vi "Example.vi"() -> ()   [LabVIEW 2014, in "Vaisala Library.lvlib" / "Vaisala.lvclass"]
doc: "Simple demonstration of how to use the Vaisala probe software."
uses:
  Vaisala.lvclass
  reusable/Session APIs/File Access/Config Data/Config Data.lvclass
  reusable/Session APIs/File Access/Config Data/Config Data.lvclass/Config Data.ctl
  Configurable Device/Configurable Device.lvclass/Configurable Device.ctl
  Data/Vaisala Data.lvclass
  Data/Vaisala Data.lvclass/Vaisala Data.ctl
  Data/Read RH.vi
  Data/Read T.vi
  Data/Read Td.vi
  reusable/Session APIs/File Access/Config Data/Accessors/Write Cfg Path.vi
  Configurable Device/Write Handle.vi
  Configurable Device/Write ID.vi
  reusable/Session APIs/File Access/Config Data/Read Array/Read String Array.vi
  reusable/Data/Read measTime.vi
  <userlib>/_Session Fwk/Session - Root.lvclass
panel:
  out "Time":timestamp format="%<%H:%M:%S%2u>T"
  out "vParams":T1(graph)
  out "error out":errorcluster
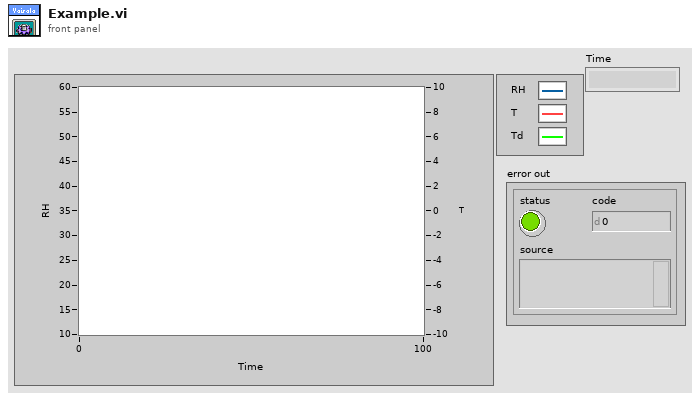
[diagram p1: front panel]
types:
  T1 = cluster{"Accessors:RH":dbl, "Accessors:T":dbl, "Accessors:Td":dbl}
  T2 = typedef "Session - Root.lvclass/Session Handle.ctl" = refnum<data-value>
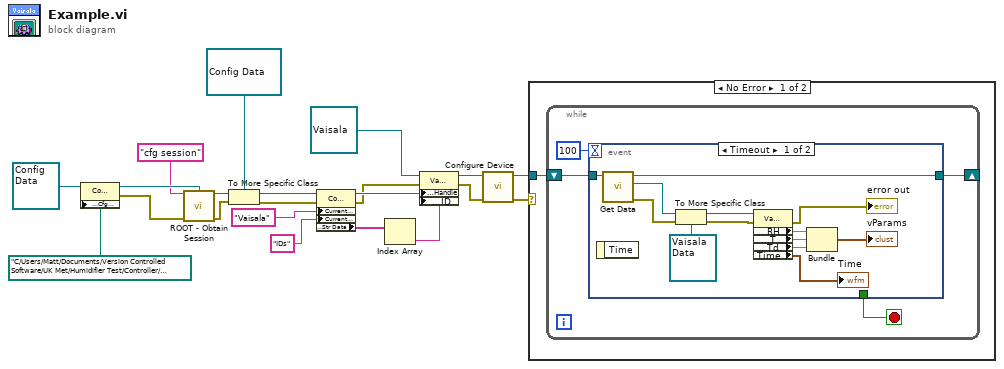
[diagram p0: block diagram]
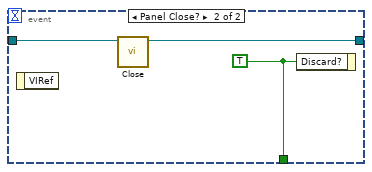
[diagram p2: hidden frame]
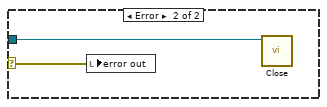
[diagram p3: hidden frame]
diagram:
  n1 = property class="Config Data"(reference=refnum<class "Config Data.lvclass"> refnum ("Config Data"), "Accessors:Cfg Path"=path "C:/Users/Matt/Documents/Version Controlled Software/UK Met/Humidifier Test/Controller/humidifier.ini" ("Cfg Path")) -> (reference out=w18:refnum<class "Config Data.lvclass">, error out=w15:errorcluster)  [unwired: 1 in]
  n2 = call <userlib>:"ROOT - Obtain Session.vi"("Session Name ()"="cfg session", "OBJ - Session"=w18, "error in (no error)"=w15) -> ("Session Handle"=w16:T2, "error out"=w14:errorcluster)  [unwired: 10 in, 1 out]
  n3 = To More Specific Class(target class=refnum<data-value> refnum ("Session Handle"), reference=w16, error in=w14) -> (specific class reference=w8:refnum<data-value>, error out=w2:errorcluster)
  n4 = property class="Config Data"(reference=w8, error in=w2, "Current Section"="Vaisala", "Current Key"="IDs") -> (reference out=w7:refnum<data-value>, error out=w1:errorcluster, "Read Array Data:Str Data"=w4:string[])
  n5 = Index Array(array=w4) -> (element=w3:string)  [unwired: 1 in]
  n6 = property class="Vaisala"(reference=refnum<class "Vaisala.lvclass"> refnum ("Vaisala"), error in=w1, "Accessors:Handle"=w7, "Accessors:ID"=w3) -> (reference out=w12:refnum<class "Vaisala.lvclass">, error out=w11:errorcluster)
  n7 = call-dynamic "Configure Device.vi"("error in"=w11, "Vaisala Probe in"=w12) -> ("error out"=w10:errorcluster, "Vaisala Probe out"=w9:refnum<class "Vaisala.lvclass">)  [unwired: 5 in, 3 out]
  n8 = case shown="No Error" w10 {
    selector: w10 -> [_ w44]
    tunnel: w9 -> [w22 w43]
    frame No Error {
      n9 = while {
        shift-right: [w25] -> _
        shift-left: w22 -> [w26]
        stop <- w24 stop-if-true
        n10 = event shown="[0] Timeout" {
          selector: _ -> [_ _]
          dyn-events: _ -> [_ _]
          timeout: 100 -> [_ _]
          tunnel: w26 -> [w39 w41]
          tunnel: [w38 w40] -> w25
          tunnel: [_ w42] -> w24
          event Timeout {
            n11 = event-data() -> ()  [unwired: 1 in, 1 out]
            n12 = call-dynamic "Get Data.vi"("Cfg Dev in"=w39) -> ("error out"=w30:errorcluster, "Data"=w37:refnum<class "Data.lvclass">, "Cfg Dev out"=w38:refnum<class "Vaisala.lvclass">)  [unwired: 8 in]
            n13 = To More Specific Class(target class=refnum<class "Vaisala Data.lvclass"> refnum ("Vaisala Library.lvlib:Vaisala Data"), reference=w37, error in=w30) -> (specific class reference=w35:refnum<class "Vaisala Data.lvclass">, error out=w29:errorcluster)
            n14 = property class="Vaisala Data"(reference=w35, error in=w29) -> (error out=→"error out":errorcluster, "Accessors:RH"=w34:dbl, "Accessors:T"=w33:dbl, "Accessors:Td"=w31:dbl, "Time"=→"Time":timestamp)  [unwired: 1 out]
            n15 = Bundle("Accessors:RH"=w34, "Accessors:T"=w33, "Accessors:Td"=w31) -> (→"vParams":T1)  [unwired: 1 in]
          }
          event Panel Close? {
            w42 = TRUE ("Discard?")
            n16 = event-data() -> ()  [unwired: 1 in, 1 out]
            n17 = call-dynamic "Close.vi"("Cfg Dev in"=w41) -> ("Cfg Dev out"=w40:refnum<class "Vaisala.lvclass">)  [unwired: 9 in, 1 out]
            n18 = event-data("Discard?"=w42) -> ()  [unwired: 1 in, 1 out]
          }
        }
      }
    }
    frame Error {
      n19 = local write "error out"(w44) -> ()
      n20 = call-dynamic "Close.vi"("Cfg Dev in"=w43) -> ()  [unwired: 9 in, 2 out]
    }
  }
